vi "Restore X & Scale Indices.vi"(5 "New Plot Style in":T1, 9 "Original Plot Style in":T1) -> (8 "Updated Plot Style out":T1)   [LabVIEW 2021, in "Graphs.lvlib"]
uses:
  Graphs.lvlib
  XY Graph/XY Graph Plot Properties.ctl
  XY Graph/XY Graph Add-Ons.lvlib
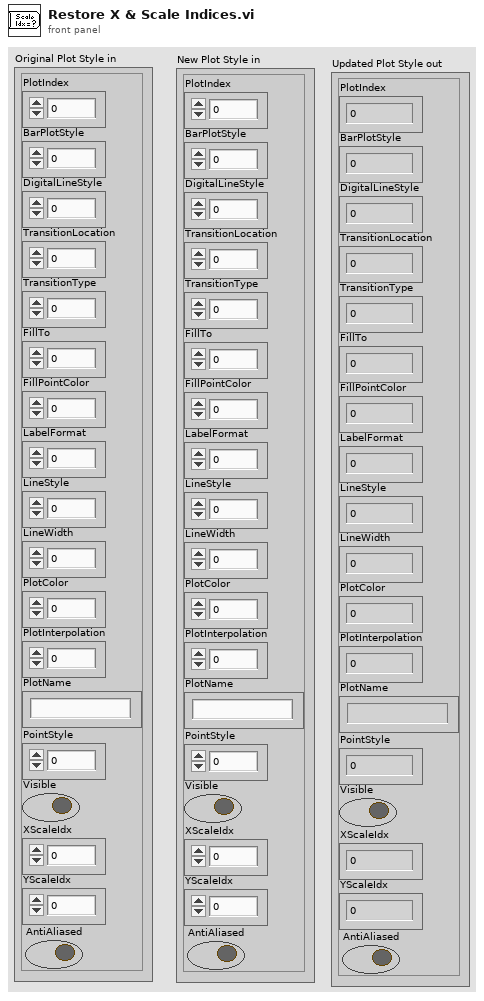
[diagram p1: front panel]
types:
  T1 = typedef "XY Graph Add-Ons.lvlib/XY Graph Plot Properties.ctl" = cluster{"PlotIndex":i32, "BarPlotStyle":u8, "DigitalLineStyle":u8, "TransitionLocation":u8, "TransitionType":u8, "FillTo":i16, "FillPointColor":u32, "LabelFormat":u8, "LineStyle":u8, "LineWidth":u8, "PlotColor":u32, "PlotInterpolation":u8, "PlotName":string, "PointStyle":u8, "Visible":bool, "XScaleIdx":u32, "YScaleIdx":u32, "AntiAliased":bool}
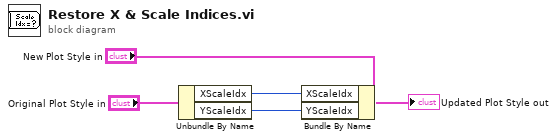
[diagram p0: block diagram]
diagram:
  n1 = Unbundle By Name("Original Plot Style in") -> ("XScaleIdx"=w2:u32, "YScaleIdx"=w1:u32)
  n2 = Bundle By Name(cluster="New Plot Style in", "XScaleIdx"=w2, "YScaleIdx"=w1) -> (→"Updated Plot Style out":T1)
